vi "Telemetry Display.vi"() -> ()   [LabVIEW 2014]
uses:
  FPGA Telemetry.ctl
  FPGA Loads and Shutdown.ctl
  Dash LED Status.ctl
  Vehicle Status/Subsystem Status.ctl
  Vehicle Status/Subsystem Status Severity.ctl
  Vehicle Status/Subsystem Status Message.ctl
  Shutdown State Machine.lvsc/State.ctl
  AIR Status.ctl
  Reason for Shutdown.ctl
  MC State Machine.lvsc/State.ctl
  CAN/MC/MC Telemetry.ctl
  CAN/MC/MC Temp 1.ctl
  CAN/MC/MC Temp 2.ctl
  CAN/MC/MC Temp 3.ctl
  CAN/MC/MC Current.ctl
  CAN/MC/MC Voltage.ctl
  CAN/MC/MC State.ctl
  CAN/Inverter States.ctl
  CAN/Inverter Run Modes.ctl
  CAN/VSM States.ctl
  CAN/MC/MC Torque.ctl
  CAN/MC/MC Position.ctl
  CAN/MC/MC Faults.ctl
  CAN/MC/MC Flux.ctl
  CAN/MC/MC Internal Voltages.ctl
  CAN/MC/MC Mod Index and Flux Weakening.ctl
  BMS Telemetry.ctl
  Vehicle Status/Remote Stop Type.ctl
  Shutdown State Machine.lvsc
  MC State Machine.lvsc
panel:
  in  "Transmit":bool
  out "Waveform Chart":dbl(graph)
  out "FPGA Fast Filename":string
  out "FPGA Slow Filename":string
  out "CAN Filename":string
  in  "New TDMS Files":bool
  out "BMS Telemetry":T1
  in  "Return to Pits":bool
  in  "Remote Stop":bool
  in  "?":bool
  in  "Telem Stop":bool
  out "MC Telemetry":T2 {"MC Faults"."MC RUN" format="%x"; "MC Faults"."MC Post" format="%x"}
  out "Telemetry":T18={"sbRIO"={"Supply Voltage (V)"=0.0, "FPGA LED"=FALSE, "Chassis Temperature"=0.0}, "Throttles"={"Throttles Consistent?"=FALSE, "Throttles In Range?"=FALSE, "Average Throttle (%)"=185.44775390625, "Throttle 2 (V)"=0.0, "Throttle 2 (%)"=-864.89453125, "Throttle 1 (V)"=15.999998092651367, "Throttle 1 (%)"=0.34765625, "Throttle 2 Max"=0.0, "Throttle 2 Min"=0.0, "Throttle 1 Max"=0.0, "Throttle 1 Min"=0.0, "Unscaled Throttle 2 Percent"=0.0, "Unscaled Throttle 1 Percent"=0.0}, "Loads & Shutdown"={"RTDS Enable"=FALSE, "TSMS In Status"=FALSE, "Positive AIR Enable"=FALSE, "cRIO Shutdown 2"=FALSE, "cRIO Shutdown 1"=FALSE, "TSMS Out Status"=FALSE, "Coolant Pump"=FALSE, "BMS OK"=FALSE, "IMD In"=FALSE, "BSPD In"=FALSE, "Brake Light Out"=FALSE, "Green LED"=enum."Off", "Yellow LED"=enum."Off", "Red LED"=enum."Off"}, "Motor Controller"={"Motor Controller Dash Switch"=FALSE, "Motor Controller Enable"=FALSE}, "Sensors"={"RL Tick Period"=0, "RR Tick Period"=0, "FR Tick Period"=0, "FL Tick Period"=0, "RR Shock (V)"=0.0, "RL Shock (V)"=0.0, "FR Shock (V)"=0.0, "FL Shock (V)"=0.0, "RR Stopped"=TRUE, "RL Stopped"=TRUE, "FR Stopped"=TRUE, "FL Stopped"=TRUE, "Steering Wheel Middle"=0.0, "Steering Wheel Angle (degrees)"=0.0, "High Current OK?"=FALSE, "Low Current OK?"=FALSE, "Rear BPS OK?"=TRUE, "Front BPS OK?"=TRUE, "Rear BP (psi)"=0.0, "Front BP (psi)"=0.0, "High Current (A)"=0.0, "Low Current (A)"=0.0, "RR State"=FALSE, "RL State"=FALSE, "FR State"=FALSE, "FL State"=FALSE, "5V Supply"=0.0}, "CPU Load"={"Total (%)"=0.0, "Time Critical (%)"=0.0, "Timed Structures (%)"=0.0, "High (%)"=0.0, "Above Normal (%)"=0.0, "Normal (%)"=0.0, "Background (%)"=0.0, "Idle (%)"=0.0, "ISR (%)"=0.0}, "Vehicle Status"={"BMS Status"={"Status Severity"=enum."Okay", "Associated Value"=0.0, "Message"=enum."ControllerTemperature", "Not OK"=FALSE}, "MC Status"={"Status Severity"=enum."Okay", "Associated Value"=0.0, "Message"=enum."ControllerTemperature", "Not OK"=FALSE}, "Shutdown Status"={"Status Severity"=enum."Okay", "Associated Value"=0.0, "Message"=enum."ControllerTemperature", "Not OK"=FALSE}, "sbRIO Status"={"Status Severity"=enum."Okay", "Associated Value"=0.0, "Message"=enum."ControllerTemperature", "Not OK"=FALSE}, "Vehicle Status"={"Status Severity"=enum."Okay", "Associated Value"=0.0, "Message"=enum."ControllerTemperature", "Not OK"=FALSE}, "Shutdown State"=enum."NI.SC.Initial", "AIR Status"=enum."Off", "Remote Return to Pits"=FALSE, "Reason for Shutdown"=enum."None", "MC State Machine Status"=enum."NI.SC.Initial"}, "iPhone HF Data"={"Accel X"=0.0, "Accel Y"=0.0, "Accel Z"=0.0, "Gyro X"=0.0, "Gyro Y"=0.0, "Gyro Z"=0.0}, "iPhone LF Data"={"Lat"=0.0, "Long"=0.0, "Speed"=0.0}} {"CPU Load"."ISR (%)" format="%#.2f"}
  # "State"
  # "Protection"
  # "Reduction"
  # "Outputs"
  # "Inputs"
  # "Torque"
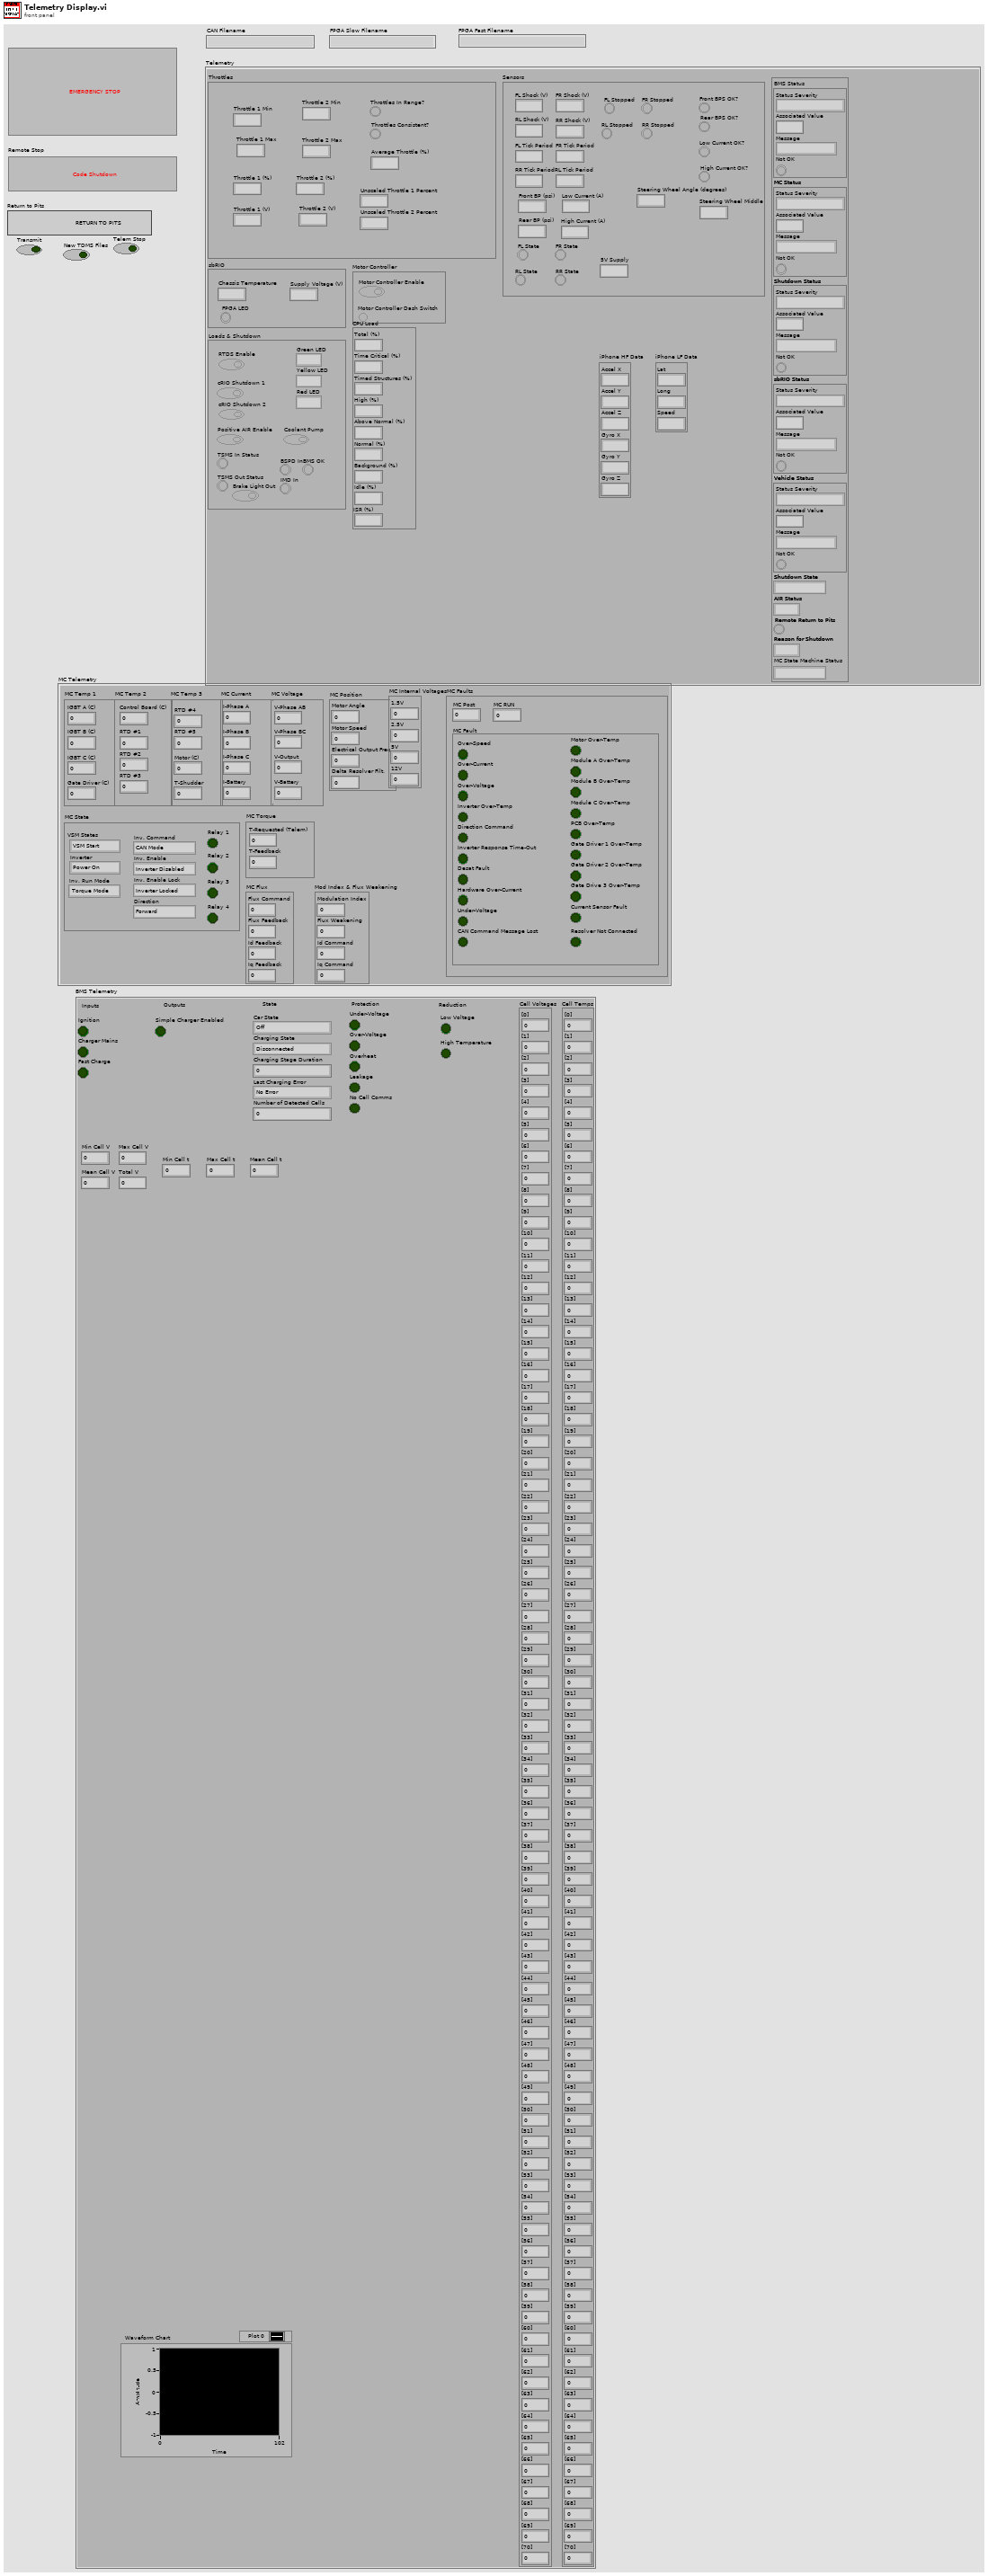
[diagram p1: front panel]
types:
  T1 = typedef "BMS Telemetry.ctl" = cluster{"Ignition":bool, "Charger Mains":bool, "Fast Charge":bool, "Simple Charger Enabled":bool, "Car State":enum16{"Off", "On, Not Charging", "Charging", "Charging Finished", "Charging Error"}, "Charging State":enum16{"Disconnected", "Pre-charging", "Main Charging", "Balancing", "Charging Finished OK", "Charging Error"}, "Charging Stage Duration":u16, "Last Charging Error":enum16{"No Error", "Cell Voltage Too Low", "No Comm from Cells so can't start", "Maximum charging stage duration expired", "No Comm from Cels so can't balande", "Cannot set balancing voltage", "Cell temps too high", "No Comms so can't determine temp", "# of Cells Mismatch", "Cells Overvoltage", "Cell Protection Event occured."}, "Number of Detected Cells":u8, "Under-Voltage":bool, "Over-Voltage":bool, "Overheat":bool, "Leakage":bool, "No Cell Comms":bool, "Low Voltage":bool, "High Temperature":bool, "Min Cell V":dbl, "Max Cell V":dbl, "Mean Cell V":dbl, "Total V":dbl, "Min Cell t":dbl, "Max Cell t":dbl, "Mean Cell t":dbl, "Cell Voltages":cluster{"[0]":dbl, "[1]":dbl, "[2]":dbl, "[3]":dbl, "[4]":dbl, "[5]":dbl, "[6]":dbl, "[7]":dbl, "[8]":dbl, "[9]":dbl, "[10]":dbl, "[11]":dbl, "[12]":dbl, "[13]":dbl, "[14]":dbl, "[15]":dbl, "[16]":dbl, "[17]":dbl, "[18]":dbl, "[19]":dbl, "[20]":dbl, "[21]":dbl, "[22]":dbl, "[23]":dbl, "[24]":dbl, "[25]":dbl, "[26]":dbl, "[27]":dbl, "[28]":dbl, "[29]":dbl, "[30]":dbl, "[31]":dbl, "[32]":dbl, "[33]":dbl, "[34]":dbl, "[35]":dbl, "[36]":dbl, "[37]":dbl, "[38]":dbl, "[39]":dbl, "[40]":dbl, "[41]":dbl, "[42]":dbl, "[43]":dbl, "[44]":dbl, "[45]":dbl, "[46]":dbl, "[47]":dbl, "[48]":dbl, "[49]":dbl, "[50]":dbl, "[51]":dbl, "[52]":dbl, "[53]":dbl, "[54]":dbl, "[55]":dbl, "[56]":dbl, "[57]":dbl, "[58]":dbl, "[59]":dbl, "[60]":dbl, "[61]":dbl, "[62]":dbl, "[63]":dbl, "[64]":dbl, "[65]":dbl, "[66]":dbl, "[67]":dbl, "[68]":dbl, "[69]":dbl, "[70]":dbl}, "Cell Temps":cluster{"[0]":dbl, "[1]":dbl, "[2]":dbl, "[3]":dbl, "[4]":dbl, "[5]":dbl, "[6]":dbl, "[7]":dbl, "[8]":dbl, "[9]":dbl, "[10]":dbl, "[11]":dbl, "[12]":dbl, "[13]":dbl, "[14]":dbl, "[15]":dbl, "[16]":dbl, "[17]":dbl, "[18]":dbl, "[19]":dbl, "[20]":dbl, "[21]":dbl, "[22]":dbl, "[23]":dbl, "[24]":dbl, "[25]":dbl, "[26]":dbl, "[27]":dbl, "[28]":dbl, "[29]":dbl, "[30]":dbl, "[31]":dbl, "[32]":dbl, "[33]":dbl, "[34]":dbl, "[35]":dbl, "[36]":dbl, "[37]":dbl, "[38]":dbl, "[39]":dbl, "[40]":dbl, "[41]":dbl, "[42]":dbl, "[43]":dbl, "[44]":dbl, "[45]":dbl, "[46]":dbl, "[47]":dbl, "[48]":dbl, "[49]":dbl, "[50]":dbl, "[51]":dbl, "[52]":dbl, "[53]":dbl, "[54]":dbl, "[55]":dbl, "[56]":dbl, "[57]":dbl, "[58]":dbl, "[59]":dbl, "[60]":dbl, "[61]":dbl, "[62]":dbl, "[63]":dbl, "[64]":dbl, "[65]":dbl, "[66]":dbl, "[67]":dbl, "[68]":dbl, "[69]":dbl, "[70]":dbl}}
  T2 = typedef "MC Telemetry.ctl" = cluster{"MC Temp 1":T3, "MC Temp 2":T4, "MC Temp 3":T5, "MC Current":T6, "MC Voltage":T7, "MC State":T8, "MC Torque":T12, "MC Position":T13, "MC Faults":T14, "MC Flux":T15, "MC Internal Voltages":T16, "Mod Index & Flux Weakening":T17}
  T3 = typedef "MC Temp 1.ctl" = cluster{"IGBT A (C)":dbl, "IGBT B (C)":dbl, "IGBT C (C)":dbl, "Gate Driver (C)":dbl}
  T4 = typedef "MC Temp 2.ctl" = cluster{"Control Board (C)":dbl, "RTD #1":dbl, "RTD #2":dbl, "RTD #3":dbl}
  T5 = typedef "MC Temp 3.ctl" = cluster{"RTD #4":dbl, "RTD #5":dbl, "Motor (C)":dbl, "T-Shudder":dbl}
  T6 = typedef "MC Current.ctl" = cluster{"I-Phase A":dbl, "I-Phase B":dbl, "I-Phase C":dbl, "I-Battery":dbl}
  T7 = typedef "MC Voltage.ctl" = cluster{"V-Phase AB":dbl, "V-Phase BC":dbl, "V-Output":dbl, "V-Battery":dbl}
  T8 = typedef "MC State.ctl" = cluster{"Inverter":T9, "Inv. Run Mode":T10, "Inv. Command":enum16{"CAN Mode", "VSM Mode"}, "Inv. Enable":enum16{"Inverter Disabled", "Inverter Enabled"}, "Inv. Enable Lock":enum16{"Inverter Locked", "Inverter Unlocked"}, "Direction":enum16{"Forward", "Reverse/Stopped"}, "VSM States":T11, "Relay 1":bool, "Relay 2":bool, "Relay 3":bool, "Relay 4":bool}
  T9 = typedef "Inverter States.ctl" = enum16{"Power On", "Stop", "Open Loop", "Closed Loop", "Wait", "Internal", "Idle Run", "Idle Stop", ""}
  T10 = typedef "Inverter Run Modes.ctl" = enum16{"Torque Mode", "Speed Mode"}
  T11 = typedef "VSM States.ctl" = enum16{"VSM Start", "Pre-Charge Init", "Pre-Charge Active", "Pre-Charge Complete", "VSM Wait", "VSM Ready", "Motor Running", "Blink Fault Code", "Shutdown in Process", "Recycle Power"}
  T12 = typedef "MC Torque.ctl" = cluster{"T-Requested (Telem)":dbl, "T-Feedback":dbl}
  T13 = typedef "MC Position.ctl" = cluster{"Motor Angle":dbl, "Motor Speed":dbl, "Electrical Output Freq.":dbl, "Delta Resolver Filt.":dbl}
  T14 = typedef "MC Faults.ctl" = cluster{"MC Fault":cluster{"Over-Speed":bool, "Over-Current":bool, "Over-Voltage":bool, "Inverter Over-Temp":bool, "Direction Command":bool, "Inverter Response Time-Out":bool, "Desat Fault":bool, "Hardware Over-Current":bool, "Under-Voltage":bool, "CAN Command Message Lost":bool, "Motor Over-Temp":bool, "Module A Over-Temp":bool, "Module B Over-Temp":bool, "Module C Over-Temp":bool, "PCB Over-Temp":bool, "Gate Driver 1 Over-Temp":bool, "Gate Driver 2 Over-Temp":bool, "Gate Drive 3 Over-Temp":bool, "Current Sensor Fault":bool, "Resolver Not Connected":bool}, "MC Post":u32, "MC RUN":u32}
  T15 = typedef "MC Flux.ctl" = cluster{"Flux Command":dbl, "Flux Feedback":dbl, "Id Feedback":dbl, "Iq Feedback":dbl}
  T16 = typedef "MC Internal Voltages.ctl" = cluster{"1.5V":dbl, "2.5V":dbl, "5V":dbl, "12V":dbl}
  T17 = typedef "MC Mod Index and Flux Weakening.ctl" = cluster{"Modulation Index":dbl, "Flux Weakening":dbl, "Id Command":dbl, "Iq Command":dbl}
  T18 = typedef "FPGA Telemetry.ctl" = cluster{"sbRIO":cluster{"Supply Voltage (V)":fxp<+/-,25,6>, "FPGA LED":bool, "Chassis Temperature":fxp<+/-,16,9>}, "Throttles":cluster{"Throttles Consistent?":bool, "Throttles In Range?":bool, "Average Throttle (%)":fxp<+/-,29,18>, "Throttle 2 (V)":fxp<+/-,24,5>, "Throttle 2 (%)":fxp<+/-,27,18>, "Throttle 1 (V)":fxp<+/-,24,5>, "Throttle 1 (%)":fxp<+/-,27,18>, "Throttle 2 Max":fxp<+,16,4>, "Throttle 2 Min":fxp<+,16,4>, "Throttle 1 Max":fxp<+,16,4>, "Throttle 1 Min":fxp<+,16,4>, "Unscaled Throttle 2 Percent":fxp<+/-,16,1>, "Unscaled Throttle 1 Percent":fxp<+/-,16,1>}, "Loads & Shutdown":T19, "Motor Controller":cluster{"Motor Controller Dash Switch":bool, "Motor Controller Enable":bool}, "Sensors":cluster{"RL Tick Period":u32, "RR Tick Period":u32, "FR Tick Period":u32, "FL Tick Period":u32, "RR Shock (V)":fxp<+/-,24,5>, "RL Shock (V)":fxp<+/-,24,5>, "FR Shock (V)":fxp<+/-,24,5>, "FL Shock (V)":fxp<+/-,24,5>, "RR Stopped":bool, "RL Stopped":bool, "FR Stopped":bool, "FL Stopped":bool, "Steering Wheel Middle":fxp<+/-,26,5>, "Steering Wheel Angle (degrees)":fxp<+/-,31,13>, "High Current OK?":bool, "Low Current OK?":bool, "Rear BPS OK?":bool, "Front BPS OK?":bool, "Rear BP (psi)":fxp<+/-,27,16>, "Front BP (psi)":fxp<+/-,27,16>, "High Current (A)":fxp<+/-,24,15>, "Low Current (A)":fxp<+/-,24,15>, "RR State":bool, "RL State":bool, "FR State":bool, "FL State":bool, "5V Supply":fxp<+/-,24,5>}, "CPU Load":cluster{"Total (%)":dbl, "Time Critical (%)":dbl, "Timed Structures (%)":dbl, "High (%)":dbl, "Above Normal (%)":dbl, "Normal (%)":dbl, "Background (%)":dbl, "Idle (%)":dbl, "ISR (%)":dbl}, "Vehicle Status":cluster{"BMS Status":T21, "MC Status":T21, "Shutdown Status":T21, "sbRIO Status":T21, "Vehicle Status":T21, "Shutdown State":T24, "AIR Status":T25, "Remote Return to Pits":bool, "Reason for Shutdown":T26, "MC State Machine Status":T27}, "iPhone HF Data":cluster{"Accel X":dbl, "Accel Y":dbl, "Accel Z":dbl, "Gyro X":dbl, "Gyro Y":dbl, "Gyro Z":dbl}, "iPhone LF Data":cluster{"Lat":dbl, "Long":dbl, "Speed":dbl}}
  T19 = typedef "FPGA Loads and Shutdown.ctl" = cluster{"RTDS Enable":bool, "TSMS In Status":bool, "Positive AIR Enable":bool, "cRIO Shutdown 2":bool, "cRIO Shutdown 1":bool, "TSMS Out Status":bool, "Coolant Pump":bool, "BMS OK":bool, "IMD In":bool, "BSPD In":bool, "Brake Light Out":bool, "Green LED":T20, "Yellow LED":T20, "Red LED":T20}
  T20 = typedef "Dash LED Status.ctl" = enum16{"Off", "Flashing", "On"}
  T21 = typedef "Subsystem Status.ctl" = cluster{"Status Severity":T22, "Associated Value":sgl, "Message":T23, "Not OK":bool}
  T22 = typedef "Subsystem Status Severity.ctl" = enum16{"Okay", "Short Warning", "Long Warning", "Return to Pits", "Error", "Danger"}
  T23 = typedef "Subsystem Status Message.ctl" = enum16{"ControllerTemperature", "MotorTemperature", "BatteryTemperature", "BatteryLowVoltage", "LVBattery", "sbRIOTemperature", "Precharge", "BSPD", "IMD", "RemoteReturnToPits", "EStopInterrupted", "NoCellComms", "MCOverSpeed", "MCOverCurrent", "MCOverVoltage", "MCInverterOverTemp", "MCDirectionCommand", "MCInverterTimeout", "MCDesatFault", "MCHWOverCurrent", "MCUnderVoltage", "MCCommandMessageLost", "MotorOverTemp", "MCModAOverTemp", "MCModBOverTemp", "MCModCOverTemp", "MCPCBOverTemp", "MCGateDrv1OverTemp", "MCDateDrv2OverTemp", "MCCurrentSensorFault", "MCResolverNotConnected", "ShutdownLatchTripped", "UnknownBMS", "RemoteEmergency"}
  T24 = typedef "Shutdown State Machine.lvsc/State.ctl" = enum16{"NI.SC.Initial", "NI.SC.History", "NI.SC.ShallowHistory", "NI.SC.Terminal", "Coolant Pump Started/AIR's On", "AIRs On", "Precharge", "TSMS Off"}
  T25 = typedef "AIR Status.ctl" = enum16{"Off", "Precharge", "On"}
  T26 = typedef "Reason for Shutdown.ctl" = enum16{"None", "BMS", "Shutdown", "sbRIO", "MC", "Remote"}
  T27 = typedef "MC State Machine.lvsc/State.ctl" = enum16{"NI.SC.Initial", "NI.SC.History", "NI.SC.ShallowHistory", "NI.SC.Terminal", "Let Current Drop then Disable AIR's", "Enabled", "Disabled"}
  T28 = typedef "Remote Stop Type.ctl" = cluster{"REMOTE STOP":bool, "REMOTE EMERGENCY STOP":bool, "Return to Pits":bool, "New TDMS Files":bool}
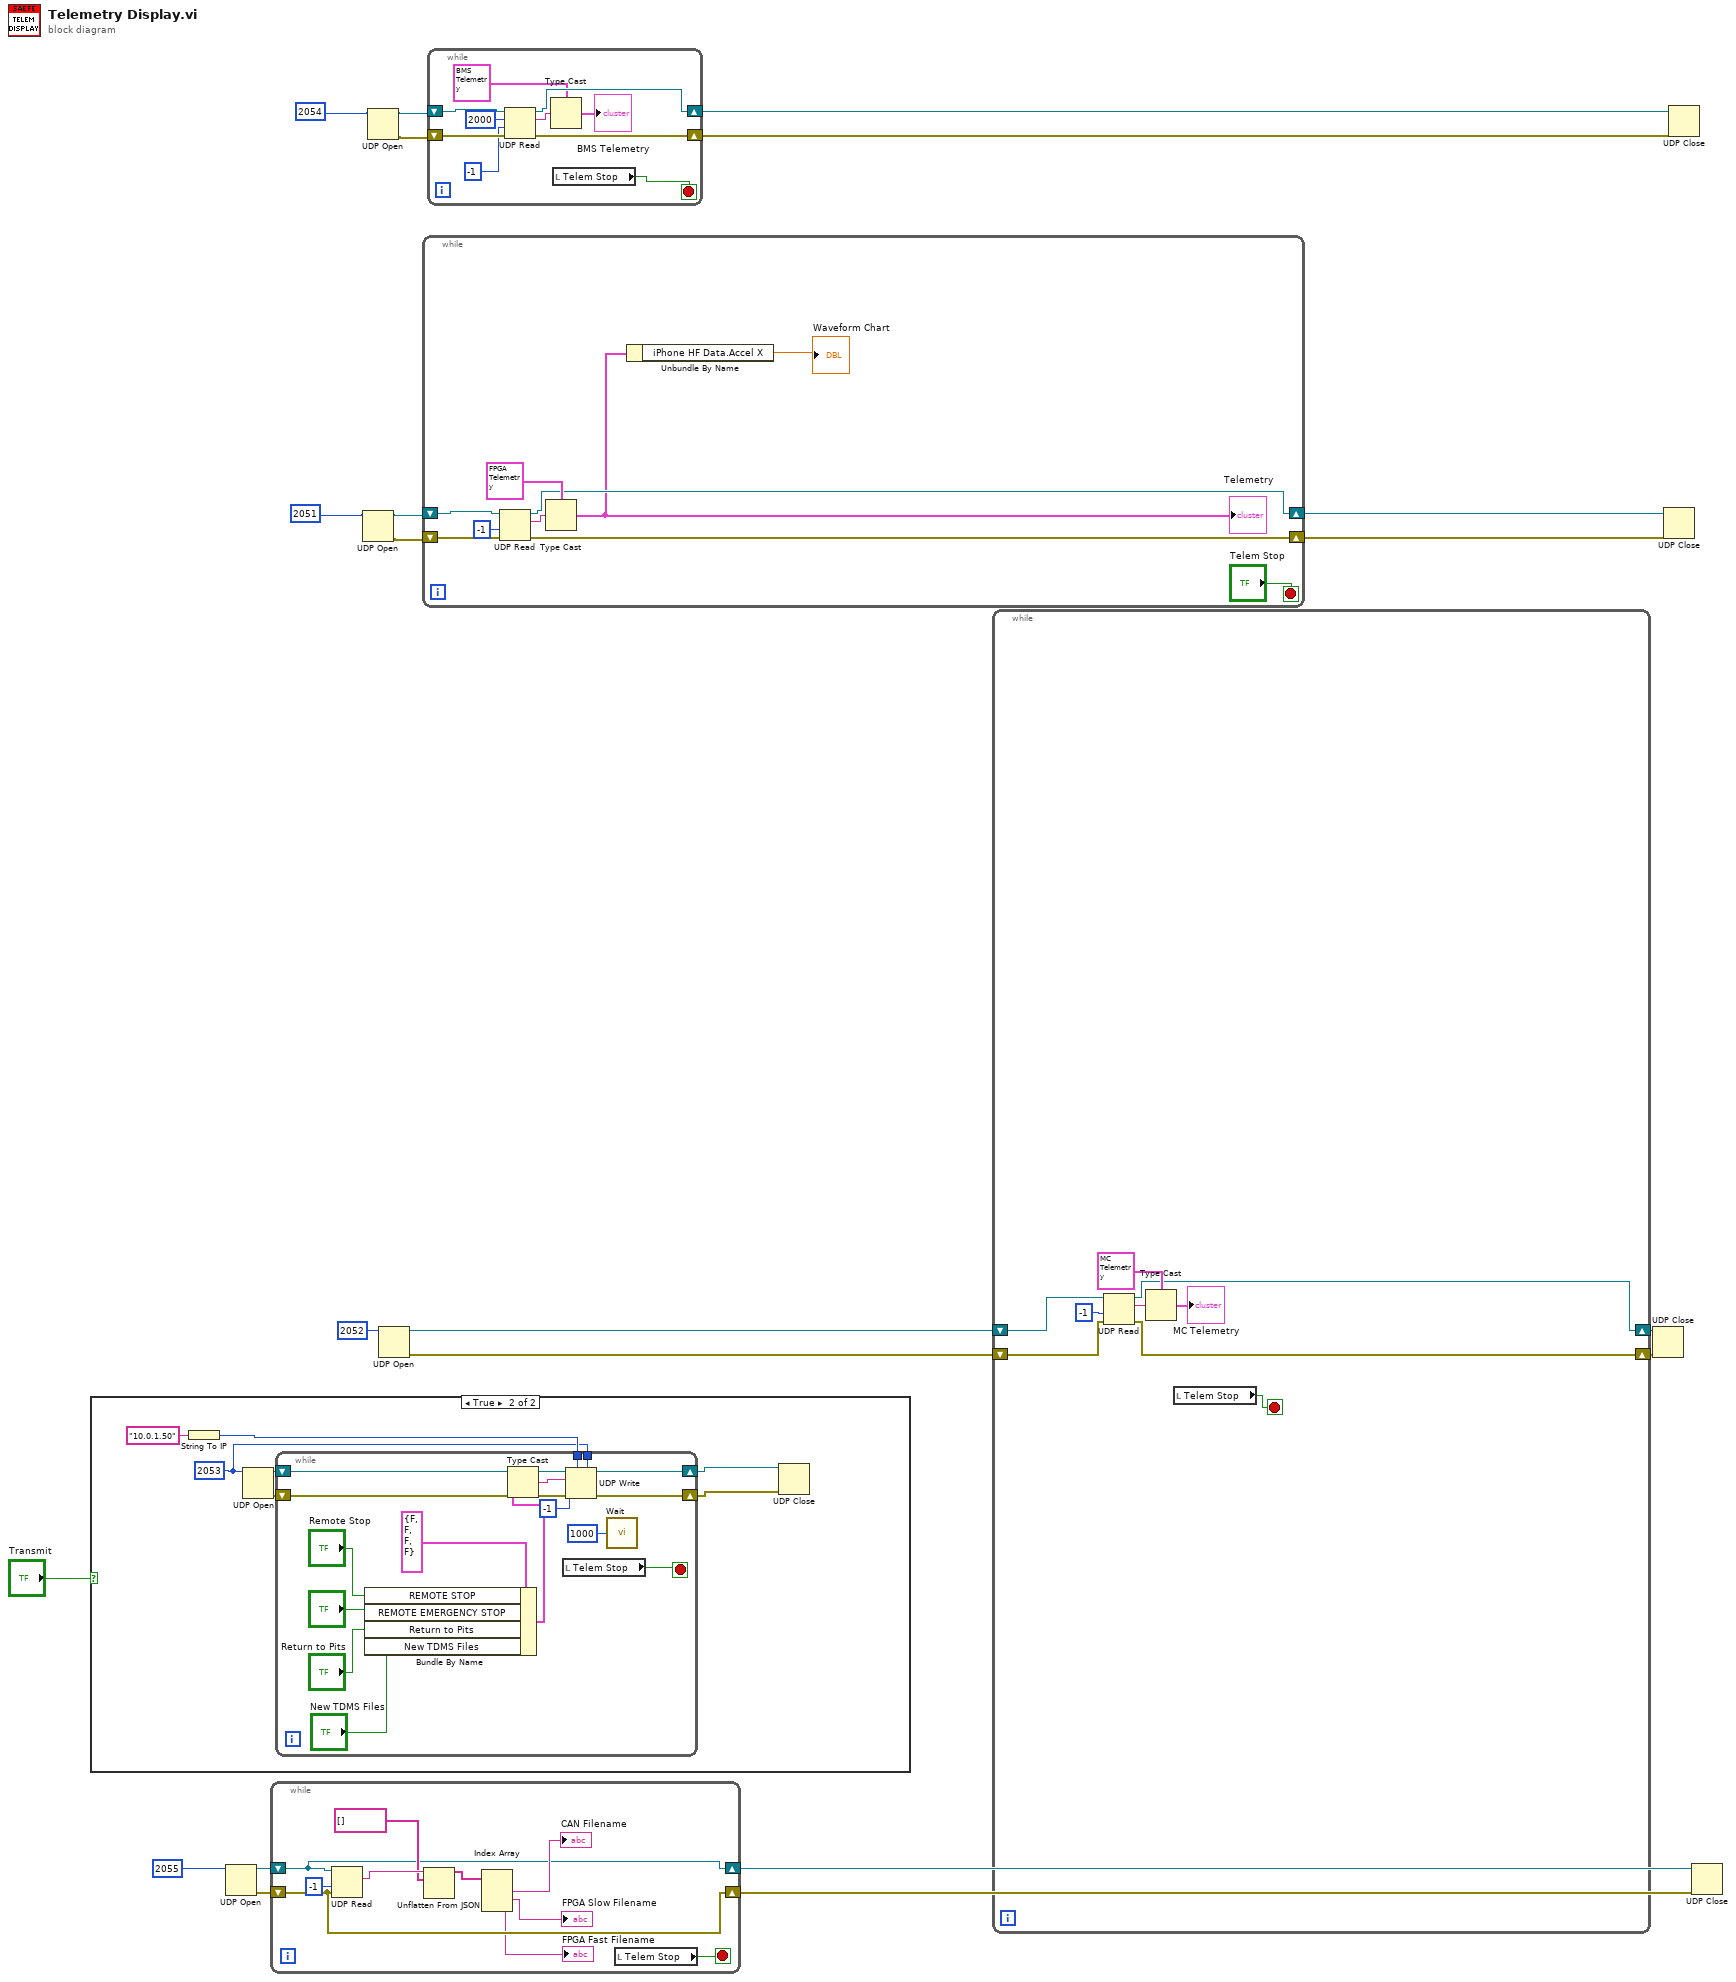
[diagram p0: block diagram]
diagram:
  n1 = case shown="True" "Transmit" {
    frame False {
    }
    frame True {
      w24 = u16 2053 ("port")
      n2 = String To IP(1:"10.0.1.50" ("name")) -> (0:w25:u32)
      n3 = UDP Open(11:w24) -> (port=w27:refnum<k16>, 0:w28:errorcluster)  [unwired: 4 in, 1 out]
      n4 = while {
        tunnel: w25 -> [w41]
        tunnel: w24 -> [w40]
        shift-right: [w39] -> w23
        shift-left: w27 -> [w42]
        shift-right: [w38] -> w22
        shift-left: w28 -> [w43]
        stop <- w36 stop-if-true
        n5 = Bundle By Name(cluster=T28 {"REMOTE STOP"=FALSE, "REMOTE EMERGENCY STOP"=FALSE, "Return to Pits"=FALSE, "New TDMS Files"=FALSE} ("Remote Signalling"), "REMOTE STOP"="Remote Stop", "REMOTE EMERGENCY STOP"="?", "Return to Pits"="Return to Pits", "New TDMS Files"="New TDMS Files") -> (w34:T28)
        n6 = Type Cast(x=w34) -> (*(type *) &x=w44:string)  [unwired: 1 in]
        n7 = local read "Telem Stop"() -> (w36:bool)
        n8 = UDP Write(address=w41, port or service name=w40, connection ID=w42, data in=w44, 8:w43, 9:-1 ("timeout ms (25000)")) -> (error out=w38:errorcluster, 3:w39:refnum<k16>)
        n9 = call "Wait"("Count(mSec)"=u32 1000) -> ()  [unwired: 1 out]
      }
      n10 = UDP Close(connection ID=w23, 8:w22) -> ()  [unwired: 2 out]
    }
  }
  n11 = UDP Open(11:u16 2055 ("port")) -> (port=w6:refnum<k16>, 0:w5:errorcluster)  [unwired: 4 in, 1 out]
  n12 = while {
    shift-right: [w49] -> w2
    shift-left: w6 -> [w49]
    shift-right: [w48] -> w3
    shift-left: w5 -> [w48]
    stop <- w50 stop-if-true
    n13 = UDP Read(connection ID=w49, timeout ms (25000)=-1, 8:w48) -> (data out=w54:string)  [unwired: 1 in, 4 out]
    n14 = Unflatten From JSON(JSON string=w54, type and defaults=string[] []) -> (value=w52:string[])  [unwired: 5 in, 1 out]
    n15 = Index Array(array=w52) -> (element #1=→"CAN Filename":string, element #2=→"FPGA Slow Filename":string, element #3=→"FPGA Fast Filename":string)  [unwired: 3 in]
    n16 = local read "Telem Stop"() -> (w50:bool)
  }
  n17 = UDP Open(11:u16 2051 ("port")) -> (port=w13:refnum<k16>, 0:w12:errorcluster)  [unwired: 4 in, 1 out]
  n18 = UDP Open(11:u16 2054 ("port")) -> (port=w8:refnum<k16>, 0:w7:errorcluster)  [unwired: 4 in, 1 out]
  n19 = UDP Open(11:u16 2052 ("port")) -> (port=w21:refnum<k16>, 0:w15:errorcluster)  [unwired: 4 in, 1 out]
  n20 = while {
    shift-right: [w61] -> w19
    shift-left: w12 -> [w62]
    shift-right: [w59] -> w18
    shift-left: w13 -> [w63]
    stop <- "Telem Stop" stop-if-true
    n21 = UDP Read(connection ID=w63, timeout ms (25000)=-1, 8:w62) -> (data out=w64:string, error out=w61:errorcluster, 3:w59:refnum<k16>)  [unwired: 1 in, 2 out]
    n22 = Type Cast(type=T18 {"sbRIO"={"Supply Voltage (V)"=0.0, "FPGA LED"=FALSE, "Chassis Temperature"=0.0}, "Throttles"={"Throttles Consistent?"=FALSE, "Throttles In Range?"=FALSE, "Average Throttle (%)"=0.0, "Throttle 2 (V)"=0.0, "Throttle 2 (%)"=0.0, "Throttle 1 (V)"=0.0, "Throttle 1 (%)"=0.0, "Throttle 2 Max"=0.0, "Throttle 2 Min"=0.0, "Throttle 1 Max"=0.0, "Throttle 1 Min"=0.0, "Unscaled Throttle 2 Percent"=0.0, "Unscaled Throttle 1 Percent"=0.0}, "Loads & Shutdown"={"RTDS Enable"=FALSE, "TSMS In Status"=FALSE, "Positive AIR Enable"=FALSE, "cRIO Shutdown 2"=FALSE, "cRIO Shutdown 1"=FALSE, "TSMS Out Status"=FALSE, "Coolant Pump"=FALSE, "BMS OK"=FALSE, "IMD In"=FALSE, "BSPD In"=FALSE, "Brake Light Out"=FALSE, "Green LED"=enum."Off", "Yellow LED"=enum."Off", "Red LED"=enum."Off"}, "Motor Controller"={"Motor Controller Dash Switch"=FALSE, "Motor Controller Enable"=FALSE}, "Sensors"={"RL Tick Period"=0, "RR Tick Period"=0, "FR Tick Period"=0, "FL Tick Period"=0, "RR Shock (V)"=0.0, "RL Shock (V)"=0.0, "FR Shock (V)"=0.0, "FL Shock (V)"=0.0, "RR Stopped"=FALSE, "RL Stopped"=FALSE, "FR Stopped"=FALSE, "FL Stopped"=FALSE, "Steering Wheel Middle"=0.0, "Steering Wheel Angle (degrees)"=0.0, "High Current OK?"=FALSE, "Low Current OK?"=FALSE, "Rear BPS OK?"=TRUE, "Front BPS OK?"=TRUE, "Rear BP (psi)"=0.0, "Front BP (psi)"=0.0, "High Current (A)"=0.0, "Low Current (A)"=0.0, "RR State"=FALSE, "RL State"=FALSE, "FR State"=FALSE, "FL State"=FALSE, "5V Supply"=0.0}, "CPU Load"={"Total (%)"=0.0, "Time Critical (%)"=0.0, "Timed Structures (%)"=0.0, "High (%)"=0.0, "Above Normal (%)"=0.0, "Normal (%)"=0.0, "Background (%)"=0.0, "Idle (%)"=0.0, "ISR (%)"=0.0}, "Vehicle Status"={"BMS Status"={"Status Severity"=enum."Okay", "Associated Value"=0.0, "Message"=enum."ControllerTemperature", "Not OK"=FALSE}, "MC Status"={"Status Severity"=enum."Okay", "Associated Value"=0.0, "Message"=enum."ControllerTemperature", "Not OK"=FALSE}, "Shutdown Status"={"Status Severity"=enum."Okay", "Associated Value"=0.0, "Message"=enum."ControllerTemperature", "Not OK"=FALSE}, "sbRIO Status"={"Status Severity"=enum."Okay", "Associated Value"=0.0, "Message"=enum."ControllerTemperature", "Not OK"=FALSE}, "Vehicle Status"={"Status Severity"=enum."Okay", "Associated Value"=0.0, "Message"=enum."ControllerTemperature", "Not OK"=FALSE}, "Shutdown State"=enum."NI.SC.Initial", "AIR Status"=enum."Off", "Remote Return to Pits"=FALSE, "Reason for Shutdown"=enum."None", "MC State Machine Status"=enum."NI.SC.Initial"}, "iPhone HF Data"={"Accel X"=0.0, "Accel Y"=0.0, "Accel Z"=0.0, "Gyro X"=0.0, "Gyro Y"=0.0, "Gyro Z"=0.0}, "iPhone LF Data"={"Lat"=0.0, "Long"=0.0, "Speed"=0.0}} ("Telemetry"), x=w64) -> (*(type *) &x=w56:T18)
    "Telemetry" <- w56
    n23 = Unbundle By Name(w56) -> ("iPhone HF Data.Accel X"=→"Waveform Chart":dbl)
  }
  n24 = while {
    shift-right: [w71] -> w11
    shift-left: w7 -> [w72]
    shift-right: [w70] -> w10
    shift-left: w8 -> [w73]
    stop <- w69 stop-if-true
    n25 = UDP Read(connection ID=w73, max size (548)=2000, timeout ms (25000)=-1 ("max size (548)"), 8:w72) -> (data out=w74:string, error out=w71:errorcluster, 3:w70:refnum<k16>)  [unwired: 2 out]
    n26 = Type Cast(type=T1 {"Ignition"=FALSE, "Charger Mains"=FALSE, "Fast Charge"=FALSE, "Simple Charger Enabled"=FALSE, "Car State"=enum."Off", "Charging State"=enum."Disconnected", "Charging Stage Duration"=0, "Last Charging Error"=enum."No Error", "Number of Detected Cells"=0, "Under-Voltage"=FALSE, "Over-Voltage"=FALSE, "Overheat"=FALSE, "Leakage"=FALSE, "No Cell Comms"=FALSE, "Low Voltage"=FALSE, "High Temperature"=FALSE, "Min Cell V"=0.0, "Max Cell V"=0.0, "Mean Cell V"=0.0, "Total V"=0.0, "Min Cell t"=0.0, "Max Cell t"=0.0, "Mean Cell t"=0.0, "Cell Voltages"={"[0]"=0.0, "[1]"=0.0, "[2]"=0.0, "[3]"=0.0, "[4]"=0.0, "[5]"=0.0, "[6]"=0.0, "[7]"=0.0, "[8]"=0.0, "[9]"=0.0, "[10]"=0.0, "[11]"=0.0, "[12]"=0.0, "[13]"=0.0, "[14]"=0.0, "[15]"=0.0, "[16]"=0.0, "[17]"=0.0, "[18]"=0.0, "[19]"=0.0, "[20]"=0.0, "[21]"=0.0, "[22]"=0.0, "[23]"=0.0, "[24]"=0.0, "[25]"=0.0, "[26]"=0.0, "[27]"=0.0, "[28]"=0.0, "[29]"=0.0, "[30]"=0.0, "[31]"=0.0, "[32]"=0.0, "[33]"=0.0, "[34]"=0.0, "[35]"=0.0, "[36]"=0.0, "[37]"=0.0, "[38]"=0.0, "[39]"=0.0, "[40]"=0.0, "[41]"=0.0, "[42]"=0.0, "[43]"=0.0, "[44]"=0.0, "[45]"=0.0, "[46]"=0.0, "[47]"=0.0, "[48]"=0.0, "[49]"=0.0, "[50]"=0.0, "[51]"=0.0, "[52]"=0.0, "[53]"=0.0, "[54]"=0.0, "[55]"=0.0, "[56]"=0.0, "[57]"=0.0, "[58]"=0.0, "[59]"=0.0, "[60]"=0.0, "[61]"=0.0, "[62]"=0.0, "[63]"=0.0, "[64]"=0.0, "[65]"=0.0, "[66]"=0.0, "[67]"=0.0, "[68]"=0.0, "[69]"=0.0, "[70]"=0.0}, "Cell Temps"={"[0]"=0.0, "[1]"=0.0, "[2]"=0.0, "[3]"=0.0, "[4]"=0.0, "[5]"=0.0, "[6]"=0.0, "[7]"=0.0, "[8]"=0.0, "[9]"=0.0, "[10]"=0.0, "[11]"=0.0, "[12]"=0.0, "[13]"=0.0, "[14]"=0.0, "[15]"=0.0, "[16]"=0.0, "[17]"=0.0, "[18]"=0.0, "[19]"=0.0, "[20]"=0.0, "[21]"=0.0, "[22]"=0.0, "[23]"=0.0, "[24]"=0.0, "[25]"=0.0, "[26]"=0.0, "[27]"=0.0, "[28]"=0.0, "[29]"=0.0, "[30]"=0.0, "[31]"=0.0, "[32]"=0.0, "[33]"=0.0, "[34]"=0.0, "[35]"=0.0, "[36]"=0.0, "[37]"=0.0, "[38]"=0.0, "[39]"=0.0, "[40]"=0.0, "[41]"=0.0, "[42]"=0.0, "[43]"=0.0, "[44]"=0.0, "[45]"=0.0, "[46]"=0.0, "[47]"=0.0, "[48]"=0.0, "[49]"=0.0, "[50]"=0.0, "[51]"=0.0, "[52]"=0.0, "[53]"=0.0, "[54]"=0.0, "[55]"=0.0, "[56]"=0.0, "[57]"=0.0, "[58]"=0.0, "[59]"=0.0, "[60]"=0.0, "[61]"=0.0, "[62]"=0.0, "[63]"=0.0, "[64]"=0.0, "[65]"=0.0, "[66]"=0.0, "[67]"=0.0, "[68]"=0.0, "[69]"=0.0, "[70]"=0.0}} ("BMS Telemetry"), x=w74) -> (*(type *) &x=→"BMS Telemetry":T1)
    n27 = local read "Telem Stop"() -> (w69:bool)
  }
  n28 = while {
    shift-right: [w80] -> w17
    shift-left: w21 -> [w82]
    shift-right: [w78] -> w16
    shift-left: w15 -> [w77]
    stop <- w79 stop-if-true
    n29 = UDP Read(connection ID=w82, timeout ms (25000)=-1, 8:w77) -> (data out=w83:string, error out=w78:errorcluster, 3:w80:refnum<k16>)  [unwired: 1 in, 2 out]
    n30 = Type Cast(type=T2 {"MC Temp 1"={"IGBT A (C)"=0.0, "IGBT B (C)"=0.0, "IGBT C (C)"=0.0, "Gate Driver (C)"=0.0}, "MC Temp 2"={"Control Board (C)"=0.0, "RTD #1"=0.0, "RTD #2"=0.0, "RTD #3"=0.0}, "MC Temp 3"={"RTD #4"=0.0, "RTD #5"=0.0, "Motor (C)"=0.0, "T-Shudder"=0.0}, "MC Current"={"I-Phase A"=0.0, "I-Phase B"=0.0, "I-Phase C"=0.0, "I-Battery"=0.0}, "MC Voltage"={"V-Phase AB"=0.0, "V-Phase BC"=0.0, "V-Output"=0.0, "V-Battery"=0.0}, "MC State"={"Inverter"=enum."Power On", "Inv. Run Mode"=enum."Torque Mode", "Inv. Command"=enum."CAN Mode", "Inv. Enable"=enum."Inverter Disabled", "Inv. Enable Lock"=enum."Inverter Locked", "Direction"=enum."Forward", "VSM States"=enum."VSM Start", "Relay 1"=FALSE, "Relay 2"=FALSE, "Relay 3"=FALSE, "Relay 4"=FALSE}, "MC Torque"={"T-Requested (Telem)"=0.0, "T-Feedback"=0.0}, "MC Position"={"Motor Angle"=0.0, "Motor Speed"=0.0, "Electrical Output Freq."=0.0, "Delta Resolver Filt."=0.0}, "MC Faults"={"MC Fault"={"Over-Speed"=FALSE, "Over-Current"=FALSE, "Over-Voltage"=FALSE, "Inverter Over-Temp"=FALSE, "Direction Command"=FALSE, "Inverter Response Time-Out"=FALSE, "Desat Fault"=FALSE, "Hardware Over-Current"=FALSE, "Under-Voltage"=FALSE, "CAN Command Message Lost"=FALSE, "Motor Over-Temp"=FALSE, "Module A Over-Temp"=FALSE, "Module B Over-Temp"=FALSE, "Module C Over-Temp"=FALSE, "PCB Over-Temp"=FALSE, "Gate Driver 1 Over-Temp"=FALSE, "Gate Driver 2 Over-Temp"=FALSE, "Gate Drive 3 Over-Temp"=FALSE, "Current Sensor Fault"=FALSE, "Resolver Not Connected"=FALSE}, "MC Post"=0, "MC RUN"=0}, "MC Flux"={"Flux Command"=0.0, "Flux Feedback"=0.0, "Id Feedback"=0.0, "Iq Feedback"=0.0}, "MC Internal Voltages"={"1.5V"=0.0, "2.5V"=0.0, "5V"=0.0, "12V"=0.0}, "Mod Index & Flux Weakening"={"Modulation Index"=0.0, "Flux Weakening"=0.0, "Id Command"=0.0, "Iq Command"=0.0}} ("MC Telemetry"), x=w83) -> (*(type *) &x=→"MC Telemetry":T2)
    n31 = local read "Telem Stop"() -> (w79:bool)
  }
  n32 = UDP Close(connection ID=w17, 8:w16) -> ()  [unwired: 2 out]
  n33 = UDP Close(connection ID=w18, 8:w19) -> ()  [unwired: 2 out]
  n34 = UDP Close(connection ID=w10, 8:w11) -> ()  [unwired: 2 out]
  n35 = UDP Close(connection ID=w2, 8:w3) -> ()  [unwired: 2 out]
